vi "Get settings chain.vi"(8 "error in (no error)":errorcluster, 11 "WaveformBase in":refnum<class "Waveform.lvclass">) -> (0 "error out":errorcluster, 1 "class name":string[](array[string]), 2 "settings":variant[](array[variant]), 3 "WaveformBase out":refnum<class "Waveform.lvclass">)   [LabVIEW 2012, in "Waveform.lvclass"]
doc: "Returns an array of variants containing the settings clusters of each class in the inheritance chain (lowest child class first), together with an array of all class names in the inheritance chain.\n\nFor classes without settings cluster, the settings chain contains empty variants."
uses:
  Waveform.lvclass
  <vilib>/Distrio/Murmex/Murmex/Murmex.lvclass
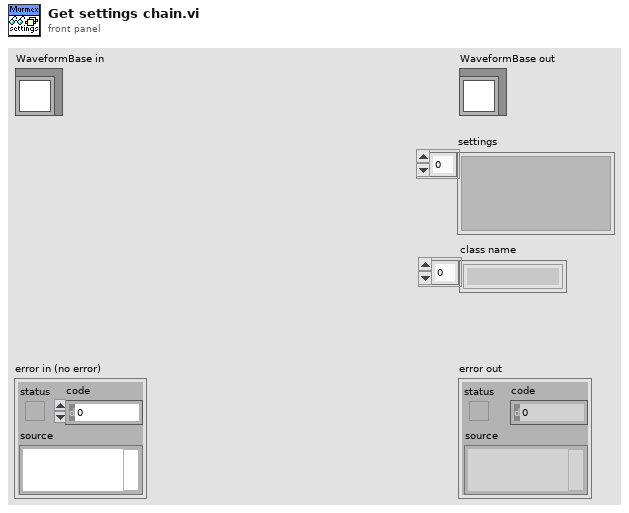
[diagram p1: front panel]
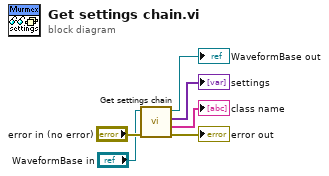
[diagram p0: block diagram]
diagram:
  n1 = call-parent "Get settings chain.vi"("error in (no error)"="error in (no error)", "MurmexBase in"="WaveformBase in") -> ("error out"=→"error out":errorcluster, "class name"=→"class name":string[], "settings"=→"settings":variant[], "MurmexBase out"=→"WaveformBase out":refnum<class "Waveform.lvclass">)  [unwired: 6 in]
